vi "toULong64Spectrum.vi"(2 "value_in":u8[](array[numeric]), 3 "dim_y":i32, 4 "dim_x":i32) -> (0 "setpoint":u64[](array[numeric]), 1 "value":u64[](array[numeric]))   [LabVIEW 2014, in "tango.lvlib"]
uses:
  tango.lvlib
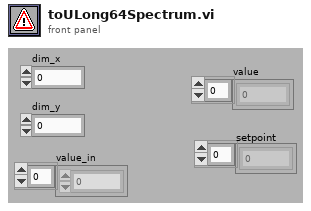
[diagram p1: front panel]
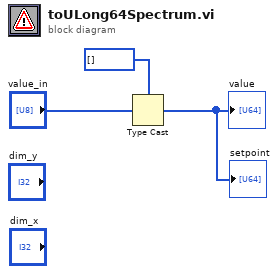
[diagram p0: block diagram]
diagram:
  n1 = Type Cast(type=u64[] [], x="value_in") -> (*(type *) &x=→"value" →"setpoint":u64[])
